vi "Autonomous new.vi"   [LabVIEW 2011]
uses:
  Team Code/Robot Global Data.vi
types:
  T1 = cluster{"Autonomous Mode":enum16{"Right", "Center", "Left", "Disable"}, "Autonomous Delay":dbl}
  T2 = enum32{"Top Hoop", "Bottom Hoop", "Left Hoop", "Right Hoop"}
  T3 = cluster{"Speed Right":dbl, "Distance Right":dbl, "Speed Left":dbl, "Distance Left":dbl}
  T4 = cluster{"Position":cluster{"X Angle":dbl, "Raw Y":dbl, "Raw X":dbl}, "Distance (ft)":dbl, "BB Angle":dbl}
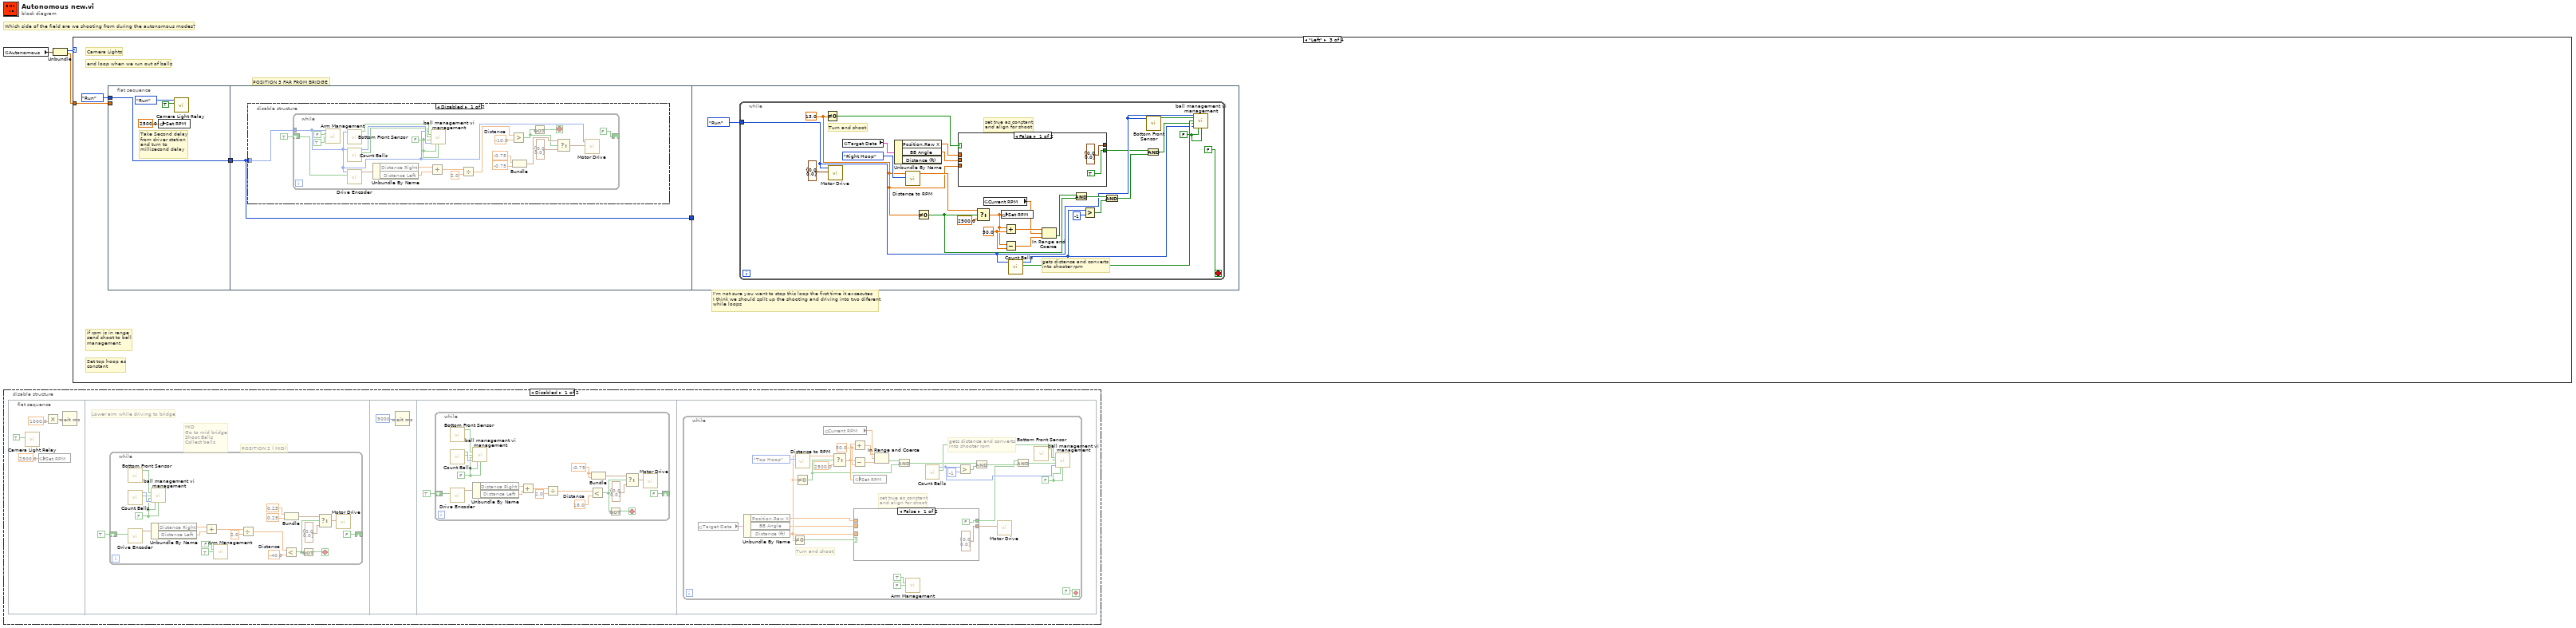
[diagram p0: block diagram]
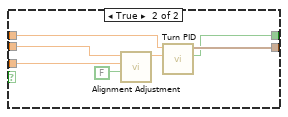
[diagram p2: hidden frame]
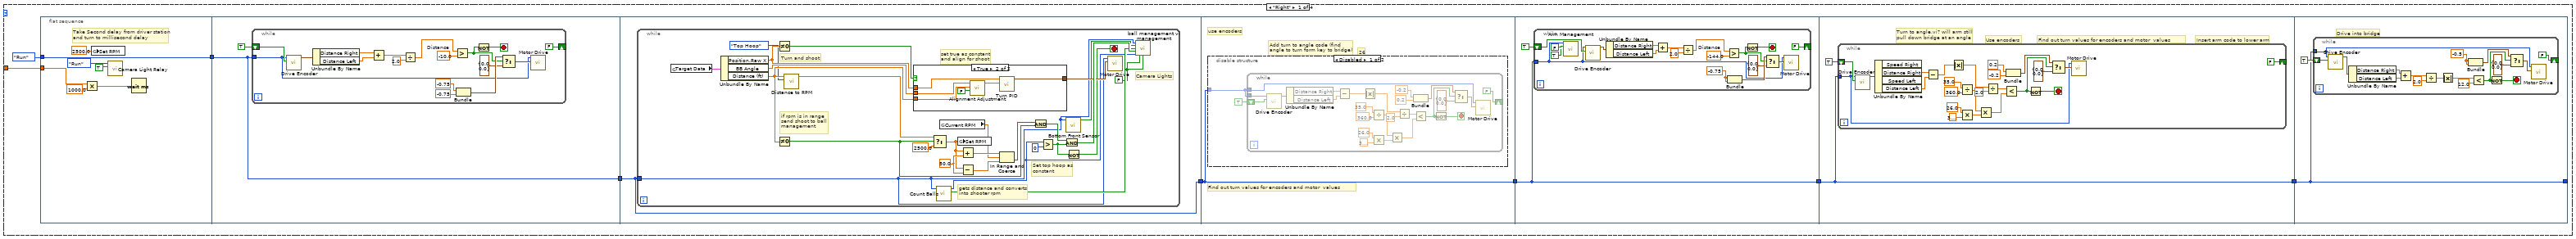
[diagram p4: hidden frame]
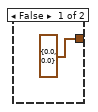
[diagram p5: hidden frame]
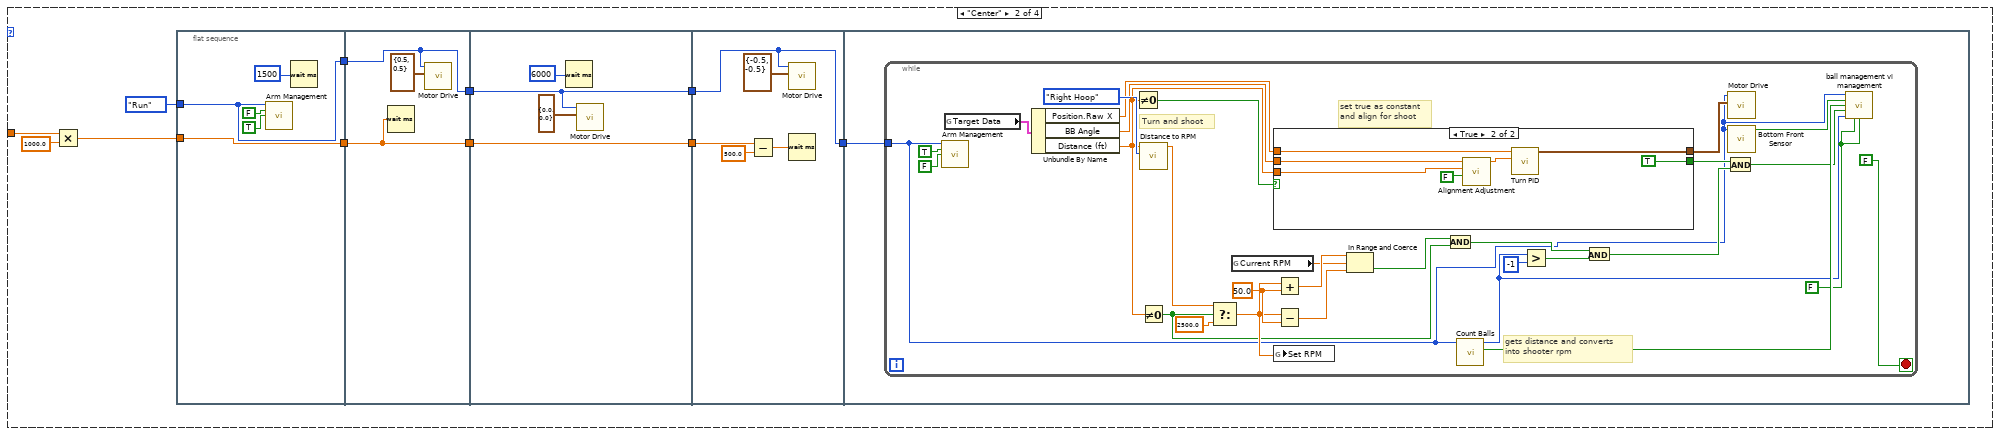
[diagram p7: hidden frame]
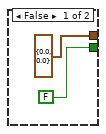
[diagram p8: hidden frame]
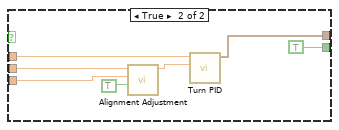
[diagram p10: hidden frame]
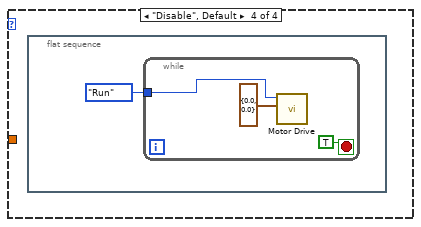
[diagram p11: hidden frame]
diagram:
  # "Which side of the field are we shooting from during the autonomous modes?"
  n1 = global read "Robot Global Data.vi" "Autonomous"() -> (w3:T1)
  n2 = disable-structure shown="Disabled" {
    frame Disabled {
      n3 = flat-sequence {
        frame #0 {
          n4 = call "Camera Light Relay.vi"("Camera Light"=TRUE) -> ()  [unwired: 11 in]
          n5 = global write "Robot Global Data.vi" "Set RPM"(2500.0 ("f")) -> ()
          n6 = Multiply(y=1000.0) -> (x*y=w7:dbl)  [unwired: 1 in]
          n7 = Wait (ms)(milliseconds to wait=w7) -> ()  [unwired: 1 out]
        }
        frame #1 {
          # "MID\nGo to mid bridge\nShoot Balls\nCollect balls"
          # "Lower arm while driving to bridge"
          # "POSITION 2 ( MID)"
          n8 = while {
            shift-right: [FALSE] -> _
            shift-left: TRUE -> [w29]
            stop <- w17 stop-if-true
            w10 = FALSE ("Manual?")
            w28 = -40.0  # Distance
            n9 = call "Bottom Front Sensor.vi"() -> ("Bottom Front"=w12:bool)  [unwired: 11 in]
            n10 = call "Count Balls.vi"() -> ("Bottom Back?"=w11:bool, "Number Of Balls"=w13:i32)  [unwired: 10 in]
            n11 = call "Drive Encoder.vi"("Reset"=w29) -> ("Encoder Values"=w30:T3)  [unwired: 10 in]
            n12 = call "ball management vi management.vi"("Bottom Front Sensor"=w12, "Bottom Back Sensor"=w11, "Shoot?"=w10, "# of Balls"=w13, "Manual Blow Hard?"=w10, "Manual SUCK-IT HARD!!!!"=w10) -> ()  [unwired: 10 in]
            n13 = Unbundle By Name(w30) -> ("Distance Right"=w27:dbl, "Distance Left"=w14:dbl)
            n14 = Add(x=w27, y=w14) -> (x+y=w25:dbl)
            n15 = call "Arm Management.vi"("Up Button"=FALSE, "Down Button"=TRUE) -> ()  [unwired: 14 in]
            n16 = Divide(x=w25, y=2.0) -> (x/y=w26:dbl)
            n17 = Bundle(0.25, 0.25) -> (w23:cluster{dbl, dbl})  [unwired: 1 in]
            n18 = Less?(x=w26, y=w28) -> (x < y?=w18:bool)
            n19 = Not(x=w18) -> (.not. x?=w17:bool)
            n20 = Select(t=w23, s=w18, f=cluster{dbl, dbl} {0.0, 0.0}) -> (s? t:f=w9:cluster{dbl, dbl})
            n21 = call "Motor Drive.vi"("Motor Input"=w9) -> ()  [unwired: 11 in]
          }
        }
        frame #2 {
          n22 = Wait (ms)(milliseconds to wait=u32 5000) -> ()  [unwired: 1 out]
        }
        frame #3 {
          n23 = while {
            shift-right: [FALSE] -> _
            shift-left: TRUE -> [w35]
            stop <- w40 stop-if-true
            w34 = FALSE ("Manual?")
            w33 = -0.75
            w50 = 18.0  # Distance
            n24 = call "Bottom Front Sensor.vi"() -> ("Bottom Front"=w37:bool)  [unwired: 11 in]
            n25 = call "Count Balls.vi"() -> ("Bottom Back?"=w36:bool, "Number Of Balls"=w38:i32)  [unwired: 10 in]
            n26 = call "Drive Encoder.vi"("Reset"=w35) -> ("Encoder Values"=w51:T3)  [unwired: 10 in]
            n27 = call "ball management vi management.vi"("Bottom Front Sensor"=w37, "Bottom Back Sensor"=w36, "Shoot?"=w34, "# of Balls"=w38, "Manual Blow Hard?"=w34, "Manual SUCK-IT HARD!!!!"=w34) -> ()  [unwired: 10 in]
            n28 = Unbundle By Name(w51) -> ("Distance Right"=w49:dbl, "Distance Left"=w39:dbl)
            n29 = Add(x=w49, y=w39) -> (x+y=w47:dbl)
            n30 = Divide(x=w47, y=2.0) -> (x/y=w48:dbl)
            n31 = Less?(x=w48, y=w50) -> (x < y?=w41:bool)
            n32 = Bundle(w33, w33) -> (w45:cluster{dbl, dbl})  [unwired: 1 in]
            n33 = Not(x=w41) -> (.not. x?=w40:bool)
            n34 = Select(t=w45, s=w41, f=cluster{dbl, dbl} {0.0, 0.0}) -> (s? t:f=w44:cluster{dbl, dbl})
            n35 = call "Motor Drive.vi"("Motor Input"=w44) -> ()  [unwired: 11 in]
          }
        }
        frame #4 {
          n36 = while {
            stop <- FALSE stop-if-true
            w78 = 50.0 ("y")
            w68 = FALSE ("Manual?")
            # "Turn and shoot"
            # "gets distance and converts \ninto shooter rpm"
            # "set true as constant\nand align for shoot"
            n37 = global read "Robot Global Data.vi" "Target Data"() -> (w72:T4)
            n38 = Unbundle By Name(w72) -> ("Position.Raw X"=w56:dbl, "BB Angle"=w54:dbl, "Distance (ft)"=w55:dbl)
            n39 = Not Equal To 0?(x=w55) -> (x != 0?=w67:bool)
            n40 = call "Distance to RPM.vi"("Distance"=w55, "Hoop"=T2."Top Hoop") -> ("Shooter RPM"=w80:dbl)  [unwired: 8 in]
            n41 = Not Equal To 0?(x=w55) -> (x != 0?=w61:bool)
            n42 = global read "Robot Global Data.vi" "Current RPM"() -> (w74:dbl)
            n43 = Select(t=w80, s=w61, f=2500.0) -> (s? t:f=w71:dbl)
            n44 = Add(x=w71, y=w78) -> (x+y=w77:dbl)
            n45 = Subtract(x=w71, y=w78) -> (x-y=w76:dbl)
            n46 = global write "Robot Global Data.vi" "Set RPM"(w71) -> ()
            n47 = case shown="False" w67 {
              tunnel: [cluster{"output":dbl, dbl} {"output"=0.0, 0.0} ("Motor Out") w88] -> w73
              tunnel: w56 -> [_ w89]
              tunnel: w54 -> [_ w87]
              tunnel: w55 -> [_ w86]
              tunnel: [FALSE ("Aligned?") w83] -> w58
              frame False {
              }
              frame True {
                n48 = call "Alignment Adjustment.vi"("Right Side of Field?"=FALSE, "Distance"=w86, "BB Angle"=w87) -> ("X Setpoint"=w85:dbl)  [unwired: 8 in]
                n49 = call "Turn PID.vi"("Setpoint X"=w85, "Current X"=w89) -> ("Aligned?"=w83:bool, "Motor Out"=w88:cluster{"output":dbl, dbl})  [unwired: 8 in]
              }
            }
            n50 = In Range and Coerce(upper limit=w77, x=w74, lower limit=w76) -> (In Range?=w62:bool)  [unwired: 1 out]
            n51 = And(x=w62, y=w61) -> (x .and. y?=w63:bool)
            n52 = call "Arm Management.vi"("Up Button"=TRUE, "Down Button"=FALSE) -> ()  [unwired: 14 in]
            n53 = call "Count Balls.vi"() -> ("Bottom Back?"=w69:bool, "Number Of Balls"=w60:i32)  [unwired: 10 in]
            n54 = Greater?(x=w60, y=-1) -> (0:w64:bool)
            n55 = And(x=w63, y=w64) -> (x .and. y?=w59:bool)
            n56 = call "Motor Drive.vi"("Motor Input"=w73) -> ()  [unwired: 11 in]
            n57 = And(x=w58, y=w59) -> (x .and. y?=w57:bool)
            n58 = call "Bottom Front Sensor.vi"() -> ("Bottom Front"=w70:bool)  [unwired: 11 in]
            n59 = call "ball management vi management.vi"("Bottom Front Sensor"=w70, "Bottom Back Sensor"=w69, "Shoot?"=w57, "# of Balls"=w60, "Manual Blow Hard?"=w68, "Manual SUCK-IT HARD!!!!"=w68) -> ()  [unwired: 10 in]
          }
        }
      }
    }
    frame Enabled {
    }
  }
  n60 = Unbundle(w3) -> ("Autonomous Mode"=w2:enum16{"Right", "Center", "Left", "Disable"}, "Autonomous Delay"=w1:dbl)
  n61 = case shown="\"Left\"" w2 {
    tunnel: w1 -> [w92 w259 w322 _]
    frame "Right" {
      n62 = flat-sequence {
        tunnel: enum16{"Init", "Run", "End"}."Run" ("Enum") -> [w104]
        tunnel: [w104] -> w91
        tunnel: w92 -> [w103]
        tunnel: w91 -> [w105]
        tunnel: [w105] -> w90
        tunnel: [w124] -> w97
        tunnel: w90 -> [w124]
        tunnel: w97 -> [w158]
        tunnel: [w158] -> w96
        tunnel: w96 -> [w186]
        tunnel: [w186] -> w95
        tunnel: [w207] -> w93
        tunnel: w95 -> [w207]
        tunnel: [w232] -> _
        tunnel: w93 -> [w232]
        frame #0 {
          # "Take Second delay from driver station\nand turn to millisecond delay"
          n63 = Multiply(x=w103, y=1000.0) -> (x*y=w102:dbl)
          n64 = global write "Robot Global Data.vi" "Set RPM"(2500.0 ("f")) -> ()
          n65 = call "Camera Light Relay.vi"("Camera Light"=TRUE, "Enum"=enum16{"Init", "Run", "End"}."Run") -> ()  [unwired: 10 in]
          n66 = Wait (ms)(milliseconds to wait=w102) -> ()  [unwired: 1 out]
        }
        frame #1 {
          n67 = while {
            shift-right: [FALSE] -> _
            shift-left: TRUE -> [w123]
            tunnel: w105 -> [w109]
            stop <- w113 stop-if-true
            w122 = -10.0  # Distance
            n68 = call "Drive Encoder.vi"("Reset"=w123, "Enum"=w109) -> ("Encoder Values"=w110:T3)  [unwired: 9 in]
            n69 = Unbundle By Name(w110) -> ("Distance Right"=w121:dbl, "Distance Left"=w112:dbl)
            n70 = Add(x=w121, y=w112) -> (x+y=w119:dbl)
            n71 = Divide(x=w119, y=2.0) -> (x/y=w120:dbl)
            n72 = Greater?(x=w120, y=w122) -> (0:w107:bool)
            n73 = Bundle(-0.75, -0.75) -> (w117:cluster{dbl, dbl})  [unwired: 1 in]
            n74 = Not(x=w107) -> (.not. x?=w113:bool)
            n75 = Select(t=w117, s=w107, f=cluster{dbl, dbl} {0.0, 0.0}) -> (s? t:f=w111:cluster{dbl, dbl})
            n76 = call "Motor Drive.vi"("Motor Input"=w111, "Enum"=w109) -> ()  [unwired: 10 in]
          }
        }
        frame #2 {
          n77 = while {
            tunnel: w124 -> [w128]
            stop <- w125 stop-if-true
            w148 = 50.0 ("y")
            w136 = FALSE ("Manual?")
            # "Turn and shoot"
            # "Camera Lights"
            # "gets distance and converts \ninto shooter rpm"
            # "if rpm is in range\nsend shoot to ball \nmanagement"
            # "Set top hoop as\nconstant"
            # "set true as constant\nand align for shoot"
            n78 = global read "Robot Global Data.vi" "Target Data"() -> (w141:T4)
            n79 = Unbundle By Name(w141) -> ("Position.Raw X"=w135:dbl, "BB Angle"=w140:dbl, "Distance (ft)"=w134:dbl)
            n80 = Not Equal To 0?(x=w135) -> (x != 0?=w133:bool)
            n81 = Not Equal To 0?(x=w134) -> (x != 0?=w129:bool)
            n82 = call "Distance to RPM.vi"("Distance"=w134, "Hoop"=T2."Top Hoop") -> ("Shooter RPM"=w150:dbl)  [unwired: 8 in]
            n83 = case shown="True" w133 {
              tunnel: [cluster{"output":dbl, dbl} {"output"=0.0, 0.0} ("Motor Out") w156] -> w142
              tunnel: w135 -> [_ w157]
              tunnel: w140 -> [_ w155]
              tunnel: w134 -> [_ w154]
              frame False {
              }
              frame True {
                n84 = call "Alignment Adjustment.vi"("Right Side of Field?"=FALSE, "Distance"=w154, "BB Angle"=w155) -> ("X Setpoint"=w153:dbl)  [unwired: 8 in]
                n85 = call "Turn PID.vi"("Setpoint X"=w153, "Current X"=w157) -> ("Motor Out"=w156:cluster{"output":dbl, dbl})  [unwired: 8 in, 1 out]
              }
            }
            n86 = Select(t=w150, s=w129, f=2500.0) -> (s? t:f=w139:dbl)
            n87 = call "Count Balls.vi"("Enum"=w128) -> ("Bottom Back?"=w137:bool, "Number Of Balls"=w126:i32)  [unwired: 9 in]
            n88 = global read "Robot Global Data.vi" "Current RPM"() -> (w143:dbl)
            n89 = global write "Robot Global Data.vi" "Set RPM"(w139) -> ()
            n90 = Add(x=w139, y=w148) -> (x+y=w147:dbl)
            n91 = Subtract(x=w139, y=w148) -> (x-y=w146:dbl)
            n92 = In Range and Coerce(upper limit=w147, x=w143, lower limit=w146) -> (In Range?=w130:bool)  [unwired: 1 out]
            n93 = And(x=w130, y=w129) -> (x .and. y?=w131:bool)
            n94 = Greater?(x=w126, y=0) -> (0:w127:bool)
            n95 = And(x=w131, y=w127) -> (x .and. y?=w144:bool)
            n96 = call "Bottom Front Sensor.vi"("Enum"=w128) -> ("Bottom Front"=w138:bool)  [unwired: 10 in]
            n97 = Not(x=w127) -> (.not. x?=w125:bool)
            n98 = call "Motor Drive.vi"("Motor Input"=w142, "Enum"=w128) -> ()  [unwired: 10 in]
            n99 = call "ball management vi management.vi"("Enum"=w128, "Bottom Front Sensor"=w138, "Bottom Back Sensor"=w137, "Shoot?"=w144, "# of Balls"=w126, "Manual Blow Hard?"=w136, "Manual SUCK-IT HARD!!!!"=w136) -> ()  [unwired: 9 in]
          }
        }
        frame #3 {
          # "26"
          # "Find out turn values for encoders and motor  values"
          # "use encoders"
          # "Add turn to angle code (find \nangle to turn form key to bridge)"
          n100 = disable-structure shown="Disabled" {
            disable-tunnel: w158 -> [w159 _]
            frame Disabled {
              n101 = while {
                shift-right: [FALSE] -> _
                shift-left: TRUE -> [w173]
                tunnel: w159 -> [w162]
                tunnel: w159 -> [w161]
                stop <- w176 stop-if-true
                n102 = call "Drive Encoder.vi"("Reset"=w173, "Enum"=w162) -> ("Encoder Values"=w185:T3)  [unwired: 9 in]
                n103 = Unbundle By Name(w185) -> ("Distance Right"=w164:dbl, "Distance Left"=w163:dbl)
                n104 = Subtract(x=w164, y=w163) -> (x-y=w184:dbl)
                n105 = Absolute Value(x=w184) -> (abs(x)=w172:dbl)
                n106 = Divide(x=35.0, y=360.0) -> (x/y=w166:dbl)
                n107 = Multiply(x=26.0, y=3.141592653589793) -> (x*y=w167:dbl)
                n108 = Multiply(x=w166, y=w167) -> (x*y=w165:dbl)
                n109 = Divide(x=w172, y=2.0) -> (x/y=w182:dbl)
                n110 = Bundle(-0.2, 0.2) -> (w181:cluster{dbl, dbl})  [unwired: 1 in]
                n111 = Less?(x=w182, y=w165) -> (x < y?=w175:bool)
                n112 = Not(x=w175) -> (.not. x?=w176:bool)
                n113 = Select(t=w181, s=w175, f=cluster{dbl, dbl} {0.0, 0.0}) -> (s? t:f=w180:cluster{dbl, dbl})
                n114 = call "Motor Drive.vi"("Motor Input"=w180, "Enum"=w161) -> ()  [unwired: 10 in]
              }
            }
            frame Enabled {
            }
          }
        }
        frame #4 {
          n115 = while {
            tunnel: w186 -> [w192]
            shift-right: [FALSE] -> _
            shift-left: TRUE -> [w195]
            stop <- w196 stop-if-true
            w189 = -0.75
            w200 = -144.0  # Distance
            n116 = call "Arm Management.vi"("Enum"=w192, "Up Button"=FALSE, "Down Button"=TRUE) -> ()  [unwired: 13 in]
            n117 = call "Drive Encoder.vi"("Reset"=w195, "Enum"=w192) -> ("Encoder Values"=w205:T3)  [unwired: 9 in]
            n118 = Unbundle By Name(w205) -> ("Distance Right"=w202:dbl, "Distance Left"=w191:dbl)
            n119 = Add(x=w202, y=w191) -> (x+y=w204:dbl)
            n120 = Divide(x=w204, y=2.0) -> (x/y=w201:dbl)
            n121 = Greater?(x=w201, y=w200) -> (0:w190:bool)
            n122 = Bundle(w189, w189) -> (w199:cluster{dbl, dbl})  [unwired: 1 in]
            n123 = Not(x=w190) -> (.not. x?=w196:bool)
            n124 = Select(t=w199, s=w190, f=cluster{dbl, dbl} {0.0, 0.0}) -> (s? t:f=w198:cluster{dbl, dbl})
            n125 = call "Motor Drive.vi"("Motor Input"=w198, "Enum"=w192) -> ()  [unwired: 10 in]
          }
        }
        frame #5 {
          # "Find out turn values for encoders and motor  values"
          # "Use encoders"
          # "Turn to angle.vi? will arm still \npull down bridge at an angle"
          # "Insert arm code to lower arm"
          n126 = while {
            shift-right: [FALSE] -> _
            shift-left: TRUE -> [w218]
            tunnel: w207 -> [w209]
            stop <- w220 stop-if-true
            n127 = call "Drive Encoder.vi"("Reset"=w218, "Enum"=w209) -> ("Encoder Values"=w231:T3)  [unwired: 9 in]
            n128 = Unbundle By Name(w231) -> ("Distance Right"=w228:dbl, "Distance Left"=w227:dbl)  [unwired: 2 out]
            n129 = Subtract(x=w228, y=w227) -> (x-y=w230:dbl)
            n130 = Absolute Value(x=w230) -> (abs(x)=w217:dbl)
            n131 = Divide(x=35.0, y=360.0) -> (x/y=w211:dbl)
            n132 = Multiply(x=26.0, y=3.141592653589793) -> (x*y=w212:dbl)
            n133 = Multiply(x=w211, y=w212) -> (x*y=w210:dbl)
            n134 = Divide(x=w217, y=2.0) -> (x/y=w226:dbl)
            n135 = Less?(x=w226, y=w210) -> (x < y?=w219:bool)
            n136 = Bundle(0.2, -0.2) -> (w225:cluster{dbl, dbl})  [unwired: 1 in]
            n137 = Not(x=w219) -> (.not. x?=w220:bool)
            n138 = Select(t=w225, s=w219, f=cluster{dbl, dbl} {0.0, 0.0}) -> (s? t:f=w224:cluster{dbl, dbl})
            n139 = call "Motor Drive.vi"("Motor Input"=w224, "Enum"=w209) -> ()  [unwired: 10 in]
          }
        }
        frame #6 {
          # "Drive into bridge"
          n140 = while {
            tunnel: w232 -> [w237]
            shift-right: [FALSE] -> _
            shift-left: TRUE -> [w238]
            stop <- w241 stop-if-true
            w236 = -0.5
            n141 = call "Drive Encoder.vi"("Reset"=w238, "Enum"=w237) -> ("Encoder Values"=w250:T3)  [unwired: 9 in]
            n142 = Unbundle By Name(w250) -> ("Distance Right"=w247:dbl, "Distance Left"=w234:dbl)
            n143 = Add(x=w247, y=w234) -> (x+y=w249:dbl)
            n144 = Divide(x=w249, y=2.0) -> (x/y=w246:dbl)
            n145 = Absolute Value(x=w246) -> (abs(x)=w235:dbl)
            n146 = Bundle(w236, w236) -> (w244:cluster{dbl, dbl})  [unwired: 1 in]
            n147 = Less?(x=w235, y=12.0 ("Distance")) -> (x < y?=w240:bool)
            n148 = Not(x=w240) -> (.not. x?=w241:bool)
            n149 = Select(t=w244, s=w240, f=cluster{dbl, dbl} {0.0, 0.0}) -> (s? t:f=w243:cluster{dbl, dbl})
            n150 = call "Motor Drive.vi"("Motor Input"=w243, "Enum"=w237) -> ()  [unwired: 10 in]
          }
        }
      }
    }
    frame "Center" {
      n151 = Multiply(x=w259, y=1000.0) -> (x*y=w258:dbl)
      n152 = flat-sequence {
        tunnel: w258 -> [w265]
        tunnel: enum16{"Init", "Run", "End"}."Run" ("Enum") -> [w266]
        tunnel: [w266] -> w257
        tunnel: [w265] -> w256
        tunnel: w257 -> [w268]
        tunnel: w256 -> [w267]
        tunnel: [w268] -> w254
        tunnel: [w267] -> w252
        tunnel: [w270] -> w255
        tunnel: w254 -> [w270]
        tunnel: [w272] -> w253
        tunnel: w252 -> [w272]
        tunnel: w255 -> [w274]
        tunnel: w253 -> [w277]
        tunnel: [w274] -> w251
        tunnel: w251 -> [w279]
        frame #0 {
          n153 = call "Arm Management.vi"("Enum"=w266, "Up Button"=FALSE, "Down Button"=TRUE) -> ()  [unwired: 13 in]
          n154 = Wait (ms)(milliseconds to wait=u32 1500) -> ()  [unwired: 1 out]
        }
        frame #1 {
          n155 = Wait (ms)(milliseconds to wait=w267) -> ()  [unwired: 1 out]
          n156 = call "Motor Drive.vi"("Motor Input"=cluster{"Left Drive":dbl, "Right Drive":dbl} {"Left Drive"=0.5, "Right Drive"=0.5}, "Enum"=w268) -> ()  [unwired: 10 in]
        }
        frame #2 {
          n157 = Wait (ms)(milliseconds to wait=u32 6000) -> ()  [unwired: 1 out]
          n158 = call "Motor Drive.vi"("Motor Input"=cluster{"Left Drive":dbl, "Right Drive":dbl} {"Left Drive"=0.0, "Right Drive"=0.0}, "Enum"=w270) -> ()  [unwired: 10 in]
        }
        frame #3 {
          n159 = Subtract(x=w277, y=500.0) -> (x-y=w275:dbl)
          n160 = call "Motor Drive.vi"("Motor Input"=cluster{"Left Drive":dbl, "Right Drive":dbl} {"Left Drive"=-0.5, "Right Drive"=-0.5}, "Enum"=w274) -> ()  [unwired: 10 in]
          n161 = Wait (ms)(milliseconds to wait=w275) -> ()  [unwired: 1 out]
        }
        frame #4 {
          n162 = while {
            tunnel: w279 -> [w280]
            stop <- FALSE stop-if-true
            w307 = 50.0 ("y")
            w297 = FALSE ("Manual?")
            # "Turn and shoot"
            # "gets distance and converts \ninto shooter rpm"
            # "set true as constant\nand align for shoot"
            n163 = call "Arm Management.vi"("Enum"=w280, "Up Button"=TRUE, "Down Button"=FALSE) -> ()  [unwired: 13 in]
            n164 = global read "Robot Global Data.vi" "Target Data"() -> (w301:T4)
            n165 = Unbundle By Name(w301) -> ("Position.Raw X"=w285:dbl, "BB Angle"=w283:dbl, "Distance (ft)"=w284:dbl)
            n166 = Not Equal To 0?(x=w284) -> (x != 0?=w296:bool)
            n167 = call "Distance to RPM.vi"("Distance"=w284, "Hoop"=T2."Right Hoop") -> ("Shooter RPM"=w309:dbl)  [unwired: 8 in]
            n168 = Not Equal To 0?(x=w284) -> (x != 0?=w290:bool)
            n169 = Select(t=w309, s=w290, f=2500.0) -> (s? t:f=w300:dbl)
            n170 = global read "Robot Global Data.vi" "Current RPM"() -> (w303:dbl)
            n171 = case shown="True" w296 {
              tunnel: [cluster{"output":dbl, dbl} {"output"=0.0, 0.0} ("Motor Out") w317] -> w302
              tunnel: w285 -> [_ w318]
              tunnel: w283 -> [_ w316]
              tunnel: w284 -> [_ w315]
              tunnel: [FALSE ("Aligned?") TRUE ("Aligned?")] -> w287
              frame False {
              }
              frame True {
                n172 = call "Alignment Adjustment.vi"("Right Side of Field?"=FALSE, "Distance"=w315, "BB Angle"=w316) -> ("X Setpoint"=w314:dbl)  [unwired: 8 in]
                n173 = call "Turn PID.vi"("Setpoint X"=w314, "Current X"=w318) -> ("Motor Out"=w317:cluster{"output":dbl, dbl})  [unwired: 8 in, 1 out]
              }
            }
            n174 = global write "Robot Global Data.vi" "Set RPM"(w300) -> ()
            n175 = Add(x=w300, y=w307) -> (x+y=w306:dbl)
            n176 = Subtract(x=w300, y=w307) -> (x-y=w305:dbl)
            n177 = In Range and Coerce(upper limit=w306, x=w303, lower limit=w305) -> (In Range?=w291:bool)  [unwired: 1 out]
            n178 = And(x=w291, y=w290) -> (x .and. y?=w292:bool)
            n179 = call "Count Balls.vi"("Enum"=w280) -> ("Bottom Back?"=w298:bool, "Number Of Balls"=w289:i32)  [unwired: 9 in]
            n180 = Greater?(x=w289, y=-1) -> (0:w293:bool)
            n181 = And(x=w292, y=w293) -> (x .and. y?=w288:bool)
            n182 = And(x=w287, y=w288) -> (x .and. y?=w286:bool)
            n183 = call "Motor Drive.vi"("Motor Input"=w302, "Enum"=w280) -> ()  [unwired: 10 in]
            n184 = call "Bottom Front Sensor.vi"("Enum"=w280) -> ("Bottom Front"=w299:bool)  [unwired: 10 in]
            n185 = call "ball management vi management.vi"("Enum"=w280, "Bottom Front Sensor"=w299, "Bottom Back Sensor"=w298, "Shoot?"=w286, "# of Balls"=w289, "Manual Blow Hard?"=w297, "Manual SUCK-IT HARD!!!!"=w297) -> ()  [unwired: 9 in]
          }
        }
      }
    }
    frame "Left" {
      # "Set top hoop as\nconstant"
      # "Camera Lights"
      # "end loop when we run out of balls"
      # "I'm not sure you want to stop this loop the first time it excecutes\nI think we should split up the shooting and driving into two diferent\nwhile loops"
      # "if rpm is in range\nsend shoot to ball \nmanagement"
      # "POSITION 3 FAR FROM BRIDGE"
      n186 = flat-sequence {
        tunnel: enum16{"Init", "Run", "End"}."Run" ("Enum") -> [w326]
        tunnel: [w326] -> w321
        tunnel: w322 -> [_]
        tunnel: w321 -> [w327]
        tunnel: [w327] -> w320
        tunnel: w320 -> [_]
        frame #0 {
          # "Take Second delay \nfrom driver station\nand turn to \nmillisecond delay"
          n187 = global write "Robot Global Data.vi" "Set RPM"(2500.0 ("f")) -> ()
          n188 = call "Camera Light Relay.vi"("Camera Light"=TRUE, "Enum"=enum16{"Init", "Run", "End"}."Run") -> ()  [unwired: 10 in]
        }
        frame #1 {
          n189 = disable-structure shown="Disabled" {
            disable-tunnel: w327 -> [w328 _]
            frame Disabled {
              n190 = while {
                shift-right: [FALSE] -> _
                shift-left: TRUE -> [w351]
                tunnel: w328 -> [w332]
                stop <- w338 stop-if-true
                w330 = FALSE ("Manual?")
                w350 = -10.0  # Distance
                n191 = call "Arm Management.vi"("Enum"=w332, "Up Button"=FALSE, "Down Button"=TRUE) -> ()  [unwired: 13 in]
                n192 = call "Bottom Front Sensor.vi"("Enum"=w332) -> ("Bottom Front"=w333:bool)  [unwired: 10 in]
                n193 = call "Count Balls.vi"("Enum"=w332) -> ("Bottom Back?"=w331:bool, "Number Of Balls"=w334:i32)  [unwired: 9 in]
                n194 = call "Drive Encoder.vi"("Reset"=w351, "Enum"=w332) -> ("Encoder Values"=w352:T3)  [unwired: 9 in]
                n195 = Unbundle By Name(w352) -> ("Distance Right"=w349:dbl, "Distance Left"=w335:dbl)
                n196 = Add(x=w349, y=w335) -> (x+y=w347:dbl)
                n197 = call "ball management vi management.vi"("Enum"=w332, "Bottom Front Sensor"=w333, "Bottom Back Sensor"=w331, "Shoot?"=w330, "# of Balls"=w334, "Manual Blow Hard?"=w330, "Manual SUCK-IT HARD!!!!"=w330) -> ()  [unwired: 9 in]
                n198 = Divide(x=w347, y=2.0) -> (x/y=w348:dbl)
                n199 = Greater?(x=w348, y=w350) -> (0:w339:bool)
                n200 = Bundle(-0.75, -0.75) -> (w345:cluster{dbl, dbl})  [unwired: 1 in]
                n201 = Not(x=w339) -> (.not. x?=w338:bool)
                n202 = Select(t=w345, s=w339, f=cluster{dbl, dbl} {0.0, 0.0}) -> (s? t:f=w342:cluster{dbl, dbl})
                n203 = call "Motor Drive.vi"("Motor Input"=w342, "Enum"=w332) -> ()  [unwired: 10 in]
              }
            }
            frame Enabled {
            }
          }
        }
        frame #2 {
          n204 = while {
            tunnel: enum16{"Init", "Run", "End"}."Run" ("Enum") -> [w362]
            stop <- FALSE stop-if-true
            w354 = 13.0 ("x")
            w379 = 50.0 ("y")
            w370 = FALSE ("Manual?")
            # "Turn and shoot"
            # "gets distance and converts \ninto shooter rpm"
            # "set true as constant\nand align for shoot"
            n205 = Not Equal To 0?(x=w354) -> (x != 0?=w369:bool)
            n206 = call "Motor Drive.vi"("Motor Input"=cluster{"Left Drive":dbl, "Right Drive":dbl} {"Left Drive"=0.0, "Right Drive"=0.0}, "Enum"=w362) -> ()  [unwired: 10 in]
            n207 = global read "Robot Global Data.vi" "Target Data"() -> (w374:T4)
            n208 = Unbundle By Name(w374) -> ("Position.Raw X"=w359:dbl, "BB Angle"=w358:dbl)  [unwired: 1 out]
            n209 = call "Distance to RPM.vi"("Distance"=w354, "Hoop"=T2."Right Hoop") -> ("Shooter RPM"=w381:dbl)  [unwired: 8 in]
            n210 = Not Equal To 0?(x=w354) -> (x != 0?=w364:bool)
            n211 = case shown="False" w369 {
              tunnel: [cluster{"output":dbl, dbl} {"output"=0.0, 0.0} ("Motor Out") w389] -> _
              tunnel: w359 -> [_ w390]
              tunnel: w358 -> [_ w388]
              tunnel: w354 -> [_ w387]
              tunnel: [TRUE ("Aligned?") TRUE ("Aligned?")] -> w361
              frame False {
              }
              frame True {
                n212 = call "Alignment Adjustment.vi"("Right Side of Field?"=TRUE, "Distance"=w387, "BB Angle"=w388) -> ("X Setpoint"=w386:dbl)  [unwired: 8 in]
                n213 = call "Turn PID.vi"("Setpoint X"=w386, "Current X"=w390) -> ("Motor Out"=w389:cluster{"output":dbl, dbl})  [unwired: 8 in, 1 out]
              }
            }
            n214 = Select(t=w381, s=w364, f=2500.0) -> (s? t:f=w373:dbl)
            n215 = global read "Robot Global Data.vi" "Current RPM"() -> (w375:dbl)
            n216 = global write "Robot Global Data.vi" "Set RPM"(w373) -> ()
            n217 = Add(x=w373, y=w379) -> (x+y=w378:dbl)
            n218 = Subtract(x=w373, y=w379) -> (x-y=w377:dbl)
            n219 = call "Count Balls.vi"("Enum"=w362) -> ("Bottom Back?"=w371:bool, "Number Of Balls"=w363:i32)  [unwired: 9 in]
            n220 = In Range and Coerce(upper limit=w378, x=w375, lower limit=w377) -> (In Range?=w356:bool)  [unwired: 1 out]
            n221 = And(x=w356, y=w364) -> (x .and. y?=w365:bool)
            n222 = Greater?(x=w363, y=-1) -> (0:w366:bool)
            n223 = And(x=w365, y=w366) -> (x .and. y?=w357:bool)
            n224 = And(x=w361, y=w357) -> (x .and. y?=w360:bool)
            n225 = call "Bottom Front Sensor.vi"("Enum"=w362) -> ("Bottom Front"=w372:bool)  [unwired: 10 in]
            n226 = call "ball management vi management.vi"("Enum"=w362, "Bottom Front Sensor"=w372, "Bottom Back Sensor"=w371, "Shoot?"=w360, "# of Balls"=w363, "Manual Blow Hard?"=w370, "Manual SUCK-IT HARD!!!!"=w370) -> ()  [unwired: 9 in]
          }
        }
      }
    }
    frame "Disable", Default {
      n227 = flat-sequence {
        frame #0 {
          n228 = while {
            tunnel: enum16{"Init", "Run", "End"}."Run" ("Enum") -> [w394]
            stop <- TRUE stop-if-true
            n229 = call "Motor Drive.vi"("Motor Input"=cluster{"Left Drive":dbl, "Right Drive":dbl} {"Left Drive"=0.0, "Right Drive"=0.0}, "Enum"=w394) -> ()  [unwired: 10 in]
          }
        }
      }
    }
  }
